vi "Inverter LUT UI.vi"(10 "Caller VI Refnum (Callee's Caller)":refnum<vi>, 11 "Main in":refnum<class "Main.lvclass">) -> (3 "Main out":refnum<class "Main.lvclass">)   [LabVIEW 2019, in "Main.lvclass"]
doc: "Developed by Kevin Thompson\nkevin@thompsonengineering.net\n\nCopyright 2020\nThompson Engineering, LLC"
uses:
  Main.lvclass
  Common/DataTypes/inverter info v2--cluster.ctl
  Common/DataTypes/inverter gain range--cluster.ctl
  Common/DataTypes/inverter offset range--cluster.ctl
  Common/DataTypes/Inverter database record v2--cluster.ctl
  Common/DataTypes/Inverter LUT v2--cluster.ctl
  <vilib>/TELLC/Dynamic CVT API/TD Dynamic CVT DVR--ref.ctl
  Main.lvclass/Main.ctl
  DataTypes/AsynCmd_Main--enum.ctl
  Accessors/Get InverterLUT Dict Ref.vi
  Accessors/Get ObjData.vi
  Accessors/Get Settings.vi
  Accessors/Set Settings.vi
  Accessors/Set InverterLUT Dict Ref.vi
  Accessors/Set CurrInverter Record.vi
  Config/Config.lvclass
  DAQ_Engine/DAQ_Engine.lvclass
  Log_Engine/Log_Engine.lvclass
panel:
  out "last updated":string="Micro < 500W"
  in  "offset range":T1={"offset max"=3000.0, "offset min"=2000.0, "offset increment"=0.0} caption="Offset Range"
  in  "gain range":T2={"gain max"=4000.0, "gain min"=3000.0, "gain increment"=100.0} caption="Gain Range"
  in  "resistance 3 phase":dbl
  in  "resistance single phase":dbl=50.0
  in  "minimum current":dbl
  in  "power level":dbl
  in  "set flag":u16(ring) items=["False", "True"]
  in  "gain actual":dbl
  in  "offset actual":dbl
  in  "inverter Info":T3
  in  "type":string="Micro < 500W"
  in  "name":string="Inverter-01"
  out "CurrRec":i32 caption="Current\nRecord Index"
  out "Total":i32 caption="Total Inverter\nRecords"
  in  "Inverter List":i32(listbox)
  in  "AddRec":bool
  in  "DeleteRec":bool
  in  "LUT File":path
  in  "Load":bool
  in  "UpdateRec":bool
  in  "Exit":bool
  # "Inverter Record"
  # "auto filled"
  # "INVERTER  DATABASE  EDITOR"
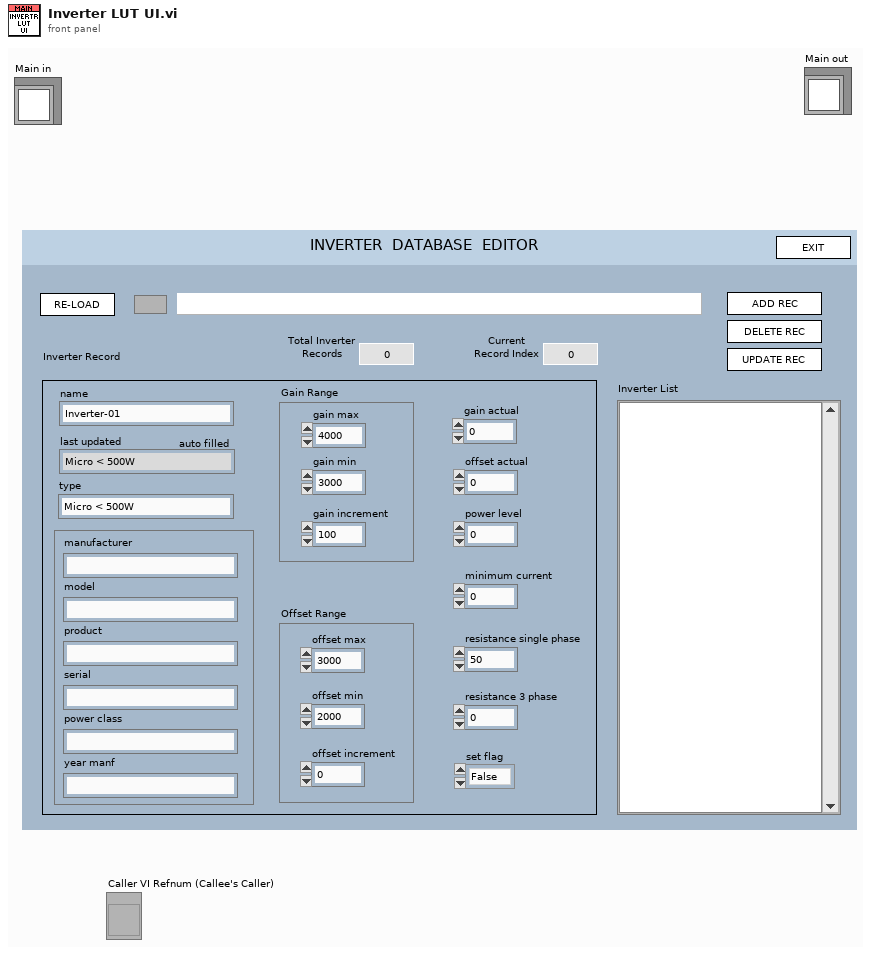
[diagram p1: front panel]
types:
  T1 = typedef "inverter offset range--cluster.ctl" = cluster{"offset max":dbl, "offset min":dbl, "offset increment":dbl}
  T2 = typedef "inverter gain range--cluster.ctl" = cluster{"gain max":dbl, "gain min":dbl, "gain increment":dbl}
  T3 = typedef "inverter info v2--cluster.ctl" = cluster{"manufacturer":string, "model":string, "product":string, "serial":string, "power class":string, "year manf":string}
  T4 = typedef "Inverter LUT v2--cluster.ctl" = cluster{"Inverter Records":T5[]}
  T5 = typedef "Inverter database record v2--cluster.ctl" = cluster{"name":string, "last updated":timestamp, "type":string, "inverter Info":T3, "gain range":T2, "offset range":T1, "gain actual":dbl, "offset actual":dbl, "power level":dbl, "minimum current":dbl, "resistance single phase":dbl, "resistance 3 phase":dbl, "set flag":u16}
  T6 = enum32{"invalid app kind", "Development System", "Run Time System", "Student Edition", "Embedded LabVIEW", "Evaluation", "Custom"}
  T7 = enum32{"Invalid", "Default", "Floating", "Floating/Auto-Hide", "Modal"}
  T8 = typedef "Main.lvclass/AsynCmd_Main--enum.ctl" = enum16{"Main.StartProcessing", "Main.StopProcessing", "Main.RefreshInverterList"}
  T9 = enum32{"Invalid", "Standard", "Closed", "Hidden", "Minimized", "Maximized"}
  T10 = typedef "TD Dynamic CVT DVR--ref.ctl" = refnum<data-value>
  T11 = cluster{"Core":cluster{"Current VI Reference":refnum<vi>, "Close Panel on Exit?":bool}, "CurrInverterRec":T5, "All Records":T5[], "Inverter Database File":path, "InverterLUT Dict":T10}
  T12 = cluster{"Current VI Reference":refnum<vi>, "Close Panel on Exit?":bool}
  T13 = typedef "Main.lvclass/ObjData--cluster.ctl" = cluster{"Settings":T14, "Public Events":T17, "Dependency":T18, "ReadData-placeholder":T19, "VISA-placeholder":refnum<visa-resource-name>, "InverterWaveformsQ":T20, "Application.TerminateProcess Event":refnum<user-event>, "RawDaqDataQ":T21, "MeasSettings":T22, "InverterDataAcqMode":T23, "DAQState Data":T24, "Private Events":T26, "InvWfmsQ-DT":T20, "DPAuxDataQ":T27, "ProcessingState":T28, "InverterInfo":T29, "CurrInverters":T5[], "InverterLUT Dict":T10, "ESR Chart Ref":refnum<vi>[], "StoreESR BLine Ref":refnum<vi>, "UseSavedESR BLine Ref":refnum<vi>, "CurrSensor":T30, "SensorLUT Dict":T10}
  T14 = typedef "Main.lvclass/Settings--cluster.ctl" = cluster{"Simulation":bool, "Signal scaling":T15[], "ESR scaling":T16[], "num readings to average":i32[], "ESR alarm threshhold (%)":i32[], "UseDummyVrms":bool, "Dummy Vrms":dbl, "Inverter Database File":path, "default Inverter (name)":string[], "Minimum Current Threshold ":dbl[], "Sensors Database File":path, "default Sensors (name)":string[]}
  T15 = typedef "Main.lvclass/Gain control.ctl" = cluster{"Iin ripple gain":dbl, "Iout ripple gain":dbl, "Iout 60Hz gain ":dbl, "Vout 60Hz gain ":dbl, "Iin ripple offest":dbl, "Iout ripple offset":dbl, "Iout 60Hz offset":dbl, "Vout 60Hz offset":dbl}
  T16 = typedef "Main.lvclass/ESR scaling--cluster.ctl" = cluster{"Gain":dbl, "Offset":dbl}
  T17 = typedef "Main.lvclass/Public Events--cluster.ctl" = cluster{"Main.AsyncCmd Event":refnum<user-event>, "Main.AsyncMsg Event":refnum<user-event>, "stop process":refnum<user-event>, "UpdateControlValue Ev":refnum<user-event>, "ProcessingStateChg Ev":refnum<user-event>}
  T18 = typedef "Main.lvclass/Dependency--cluster.ctl" = cluster{"Config":refnum<class "Config.lvclass">, "DAQ":refnum<class "DAQ_Engine.lvclass">, "Log_Engine":refnum<class "Log_Engine.lvclass">}
  T19 = typedef "Main.lvclass/Read Data--cluster.ctl" = cluster{"Data":dbl}
  T20 = typedef "InverterWaveforms--QRef.ctl" = refnum<queue>
  T21 = typedef "RawDAQDataQRef--cluster.ctl" = refnum<queue>
  T22 = typedef "Measurement Config--cluster.ctl" = cluster{"Data Rate 9775":dbl, "Data Rate 9215":dbl, "Samples RMS 9215":u32, "Samples RMS 9775":u32}
  T23 = typedef "Acquisition Mode--cluster.ctl" = enum16{"3phase", "Single"}
  T24 = typedef "DAQ_Engine.lvclass/DAQStateEvData--cluster.ctl" = cluster{"DAQState":T25, "vData":variant}
  T25 = typedef "DAQState--enum.ctl" = enum16{"Unknown", "Stopped", "Running", "Error"}
  T26 = typedef "Main.lvclass/Private Events--cluster.ctl" = cluster{"PrivateAsync Ev":refnum<user-event>}
  T27 = typedef "DataProcAuxDat--Qref.ctl" = refnum<queue>
  T28 = typedef "Main.lvclass/ProcessingState--enum.ctl" = enum16{"Idle", "Starting", "Running", "Done", "Error"}
  T29 = typedef "InverterInfo--cluster.ctl" = cluster{"Inverter ID":string}
  T30 = typedef "Sensor LUT--cluster.ctl" = T31[]
  T31 = typedef "Sensor database record--cluster.ctl" = cluster{"name":string, "last updated":timestamp, "manufacturer":string, "model":string, "Sensitivity index":dbl, "Sensor Ranges":T32}
  T32 = typedef "Sensor ranges--cluster.ctl" = cluster{"Max.VOut.RMS (V)":dbl, "Max.Out.Peak (V)":dbl, "Sensitivity (mV/A)":dbl, "Max.IOut.RMS(A)":dbl, "Min.IOut.RMS(A)":dbl}
  T33 = enum16{"Left Button", "Center Button", "Right Button", "Window Close"}
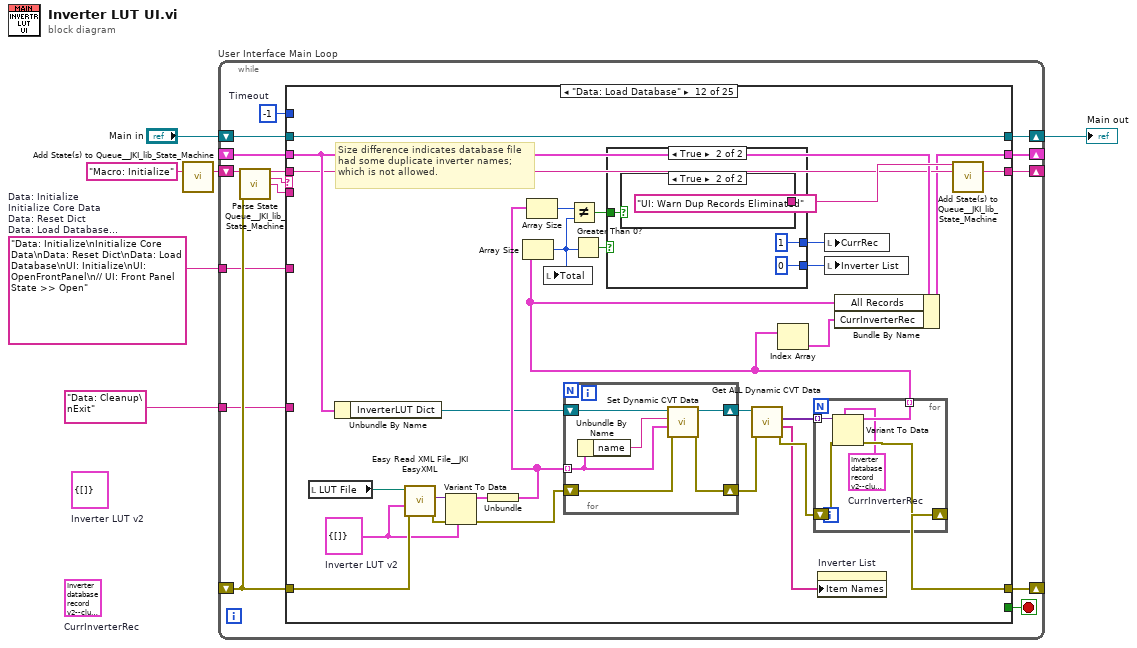
[diagram p0: block diagram]
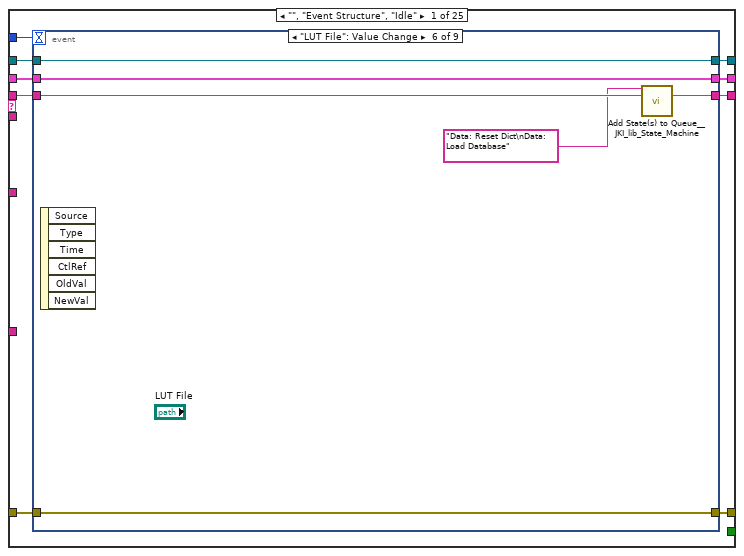
[diagram p2: hidden frame]
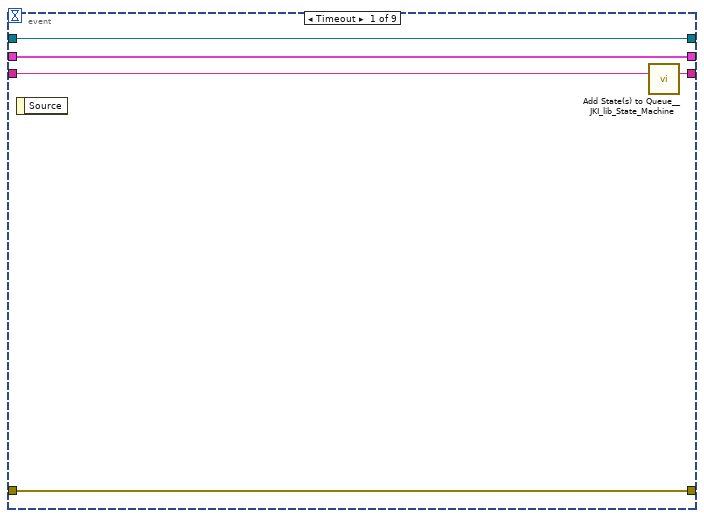
[diagram p3: hidden frame]
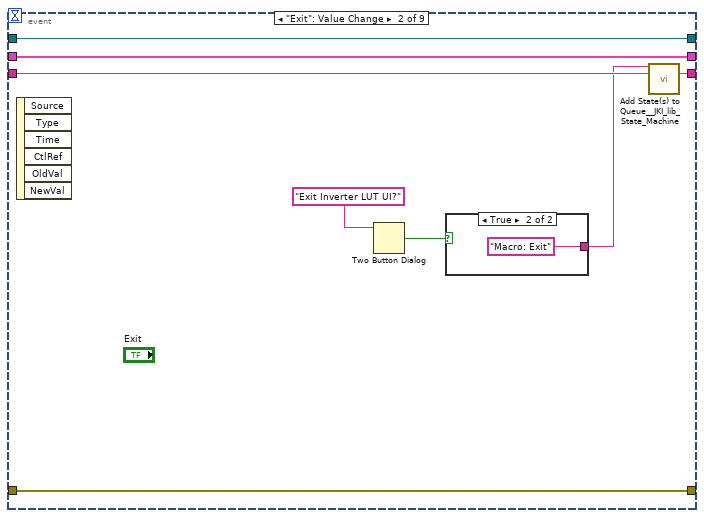
[diagram p4: hidden frame]
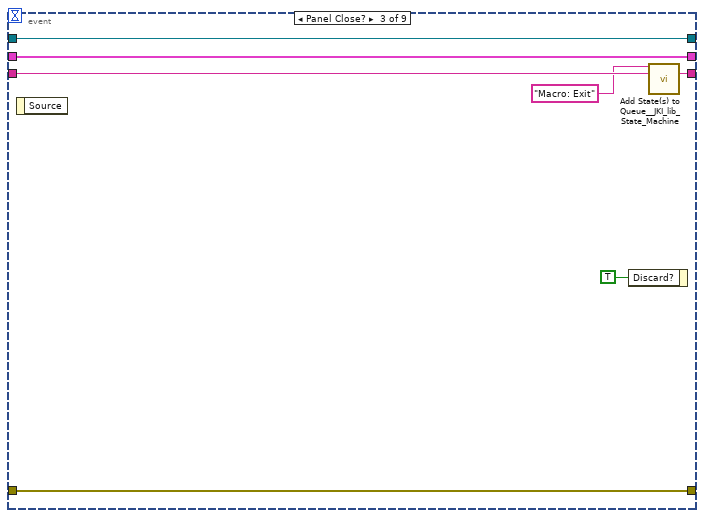
[diagram p6: hidden frame]
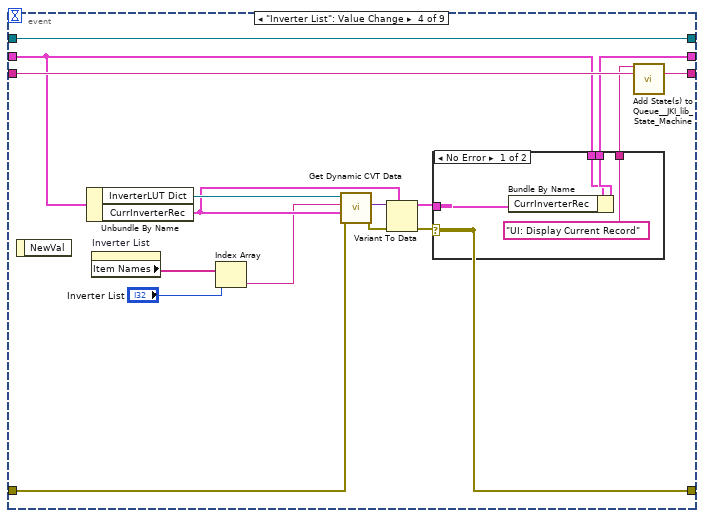
[diagram p7: hidden frame]
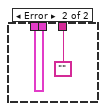
[diagram p8: hidden frame]
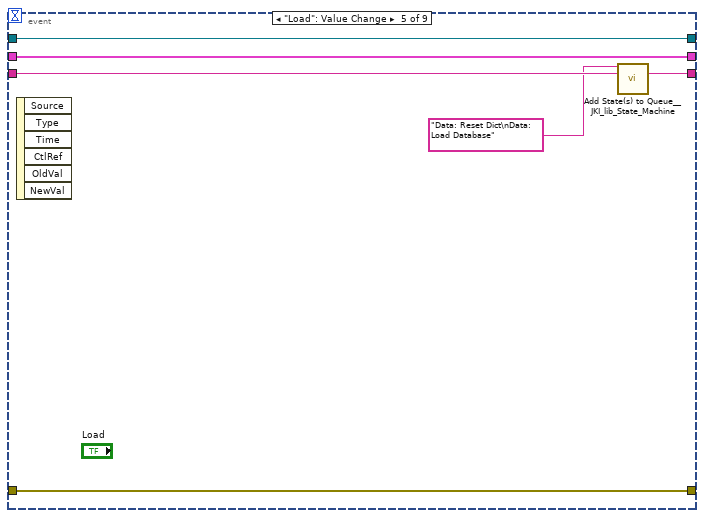
[diagram p9: hidden frame]
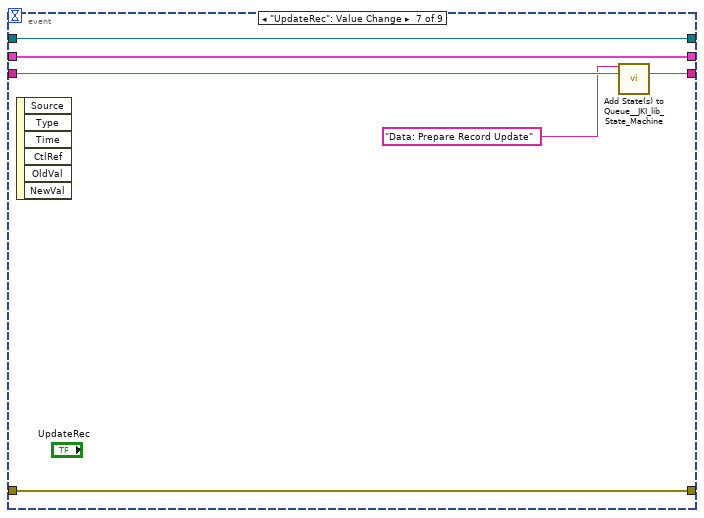
[diagram p10: hidden frame]
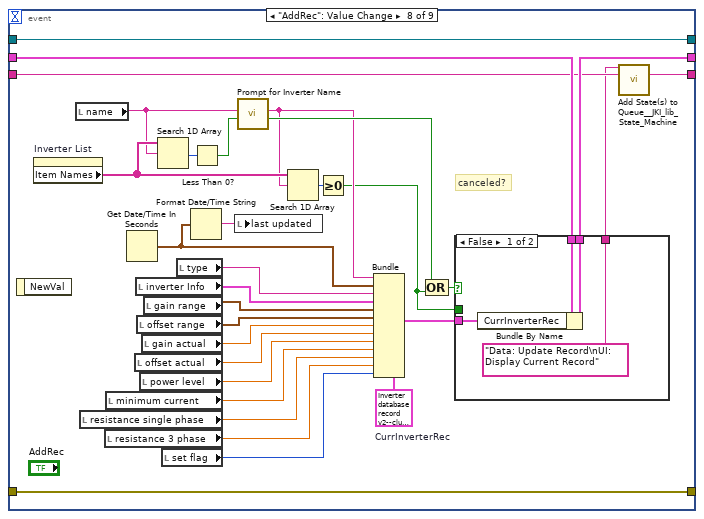
[diagram p11: hidden frame]
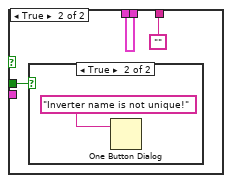
[diagram p12: hidden frame]
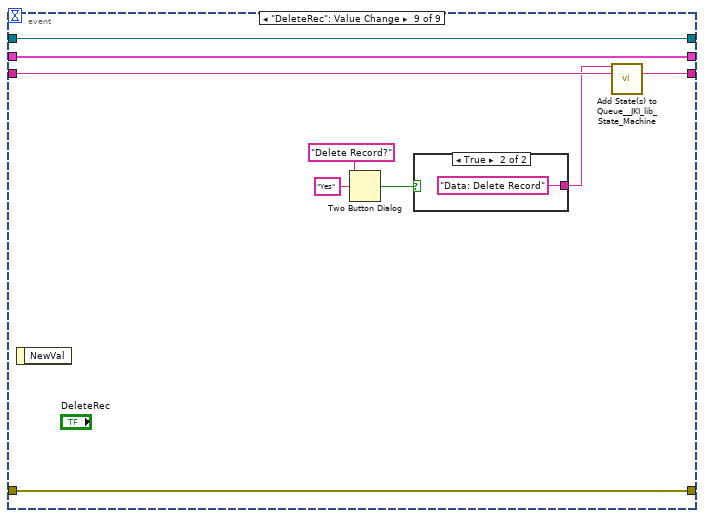
[diagram p14: hidden frame]
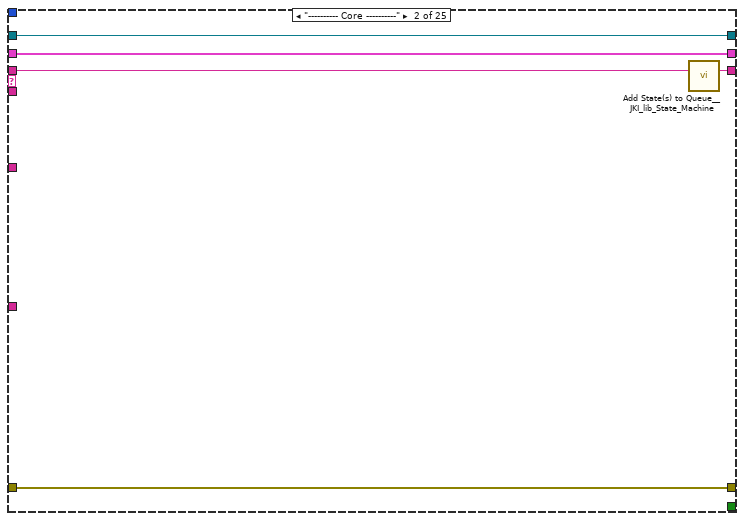
[diagram p16: hidden frame]
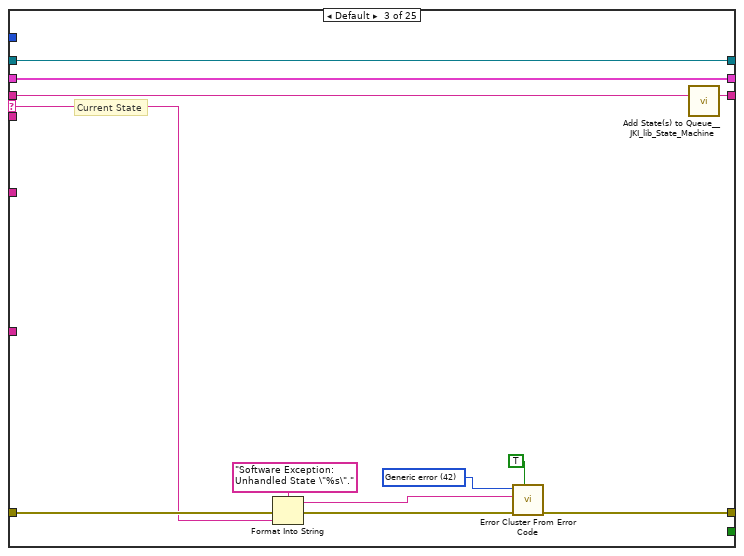
[diagram p17: hidden frame]
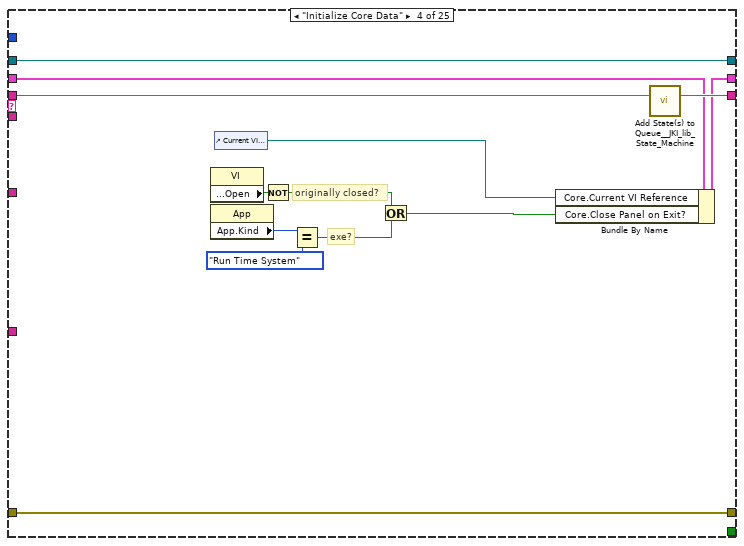
[diagram p18: hidden frame]
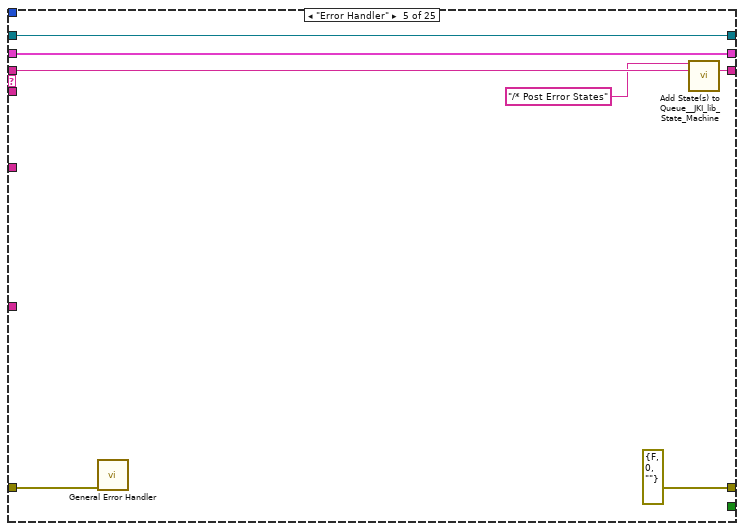
[diagram p19: hidden frame]
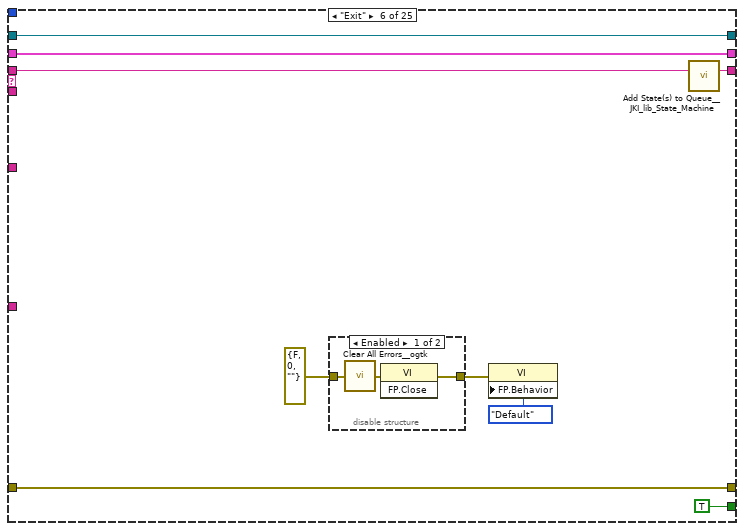
[diagram p20: hidden frame]
diagram:
  (unwired) T4 {"Inverter Records"=[]}  # Inverter LUT v2
  (unwired) T5 {"name"="", "last updated"=timestamp(0 s since 1904-01-01), "type"="", "inverter Info"={"manufacturer"="", "model"="", "product"="", "serial"="", "power class"="", "year manf"=""}, "gain range"={"gain max"=0.0, "gain min"=0.0, "gain increment"=0.0}, "offset range"={"offset max"=0.0, "offset min"=0.0, "offset increment"=0.0}, "gain actual"=0.0, "offset actual"=0.0, "power level"=0.0, "minimum current"=0.0, "resistance single phase"=0.0, "resistance 3 phase"=0.0, "set flag"=0}  # CurrInverterRec
  w4 = "Data: Initialize\nInitialize Core Data\nData: Reset Dict\nData: Load Database\nUI: Initialize\nUI: OpenFrontPanel\n// UI: Front Panel State >> Open"  # Data: Initialize Initialize Core Data Data: Reset Dict Data: Load Database UI: Initialize UI: OpenFrontPanel // UI: Front Panel State >> Open
  n1 = call <vilib>:"Add State(s) to Queue__JKI_lib_State_Machine.vi"("State(s) in (\"\")"="Macro: Initialize") -> ("States Out"=w6:string)  [unwired: 14 in]
  n2 = while "User Interface Main Loop" {
    shift-right: [w14] -> _
    shift-left: _ -> [w13]
    shift-right: [w17] -> _
    shift-left: _ -> [w11]
    shift-right: [w16] -> _
    shift-left: w6 -> [w18]
    tunnel: w4 -> [w10]
    tunnel: "Data: Cleanup\nExit" -> [w9]
    shift-right: [w7] -> w1
    shift-left: "Main in" -> [w8]
    stop <- w15 stop-if-true
    w12 = -1  # Timeout
    n3 = call <vilib>:"Parse State Queue__JKI_lib_State_Machine.vi"("State Queue"=w18, "Error In (no error)"=w11) -> ("Remaining States"=w20:string, "Current State"=w21:string, "Arguments"=w19:string)  [unwired: 11 in]
    n4 = case shown="\"Data: Load Database\"" w21 {
      selector: w21 -> [_ _ w147 _ _ _ _ _ _ _ _ _ _ _ _ _ _ _ _ _ _ _ _ _ _]
      tunnel: w20 -> [w30 w145 w151 w170 w177 w186 w195 w224 w237 w258 w288 w299 w363 w386 w401 w411 w436 w459 w479 w486 w498 w525 w531 w542 w547]
      tunnel: w19 -> [_ _ _ _ _ _ _ _ _ _ _ _ _ _ _ _ _ _ _ w481 w492 _ _ _ _]
      tunnel: w13 -> [w28 w142 w149 w161 w174 w184 w192 w218 w235 w248 w286 w306 _ w374 w398 w408 w422 w444 w471 w484 w494 w522 w528 w539 w544]
      tunnel: [w27 w143 w153 w167 errorcluster {"status"=FALSE, "code"=0, "source"=""} ("error out") w183 w193 w222 w233 w243 w277 w301 w360 w382 w399 w409 w434 w457 w461 w482 w495 w523 w529 w540 w545] -> w17
      tunnel: w11 -> [w26 w143 w152 w167 w173 w183 w193 w222 w232 w242 w283 w302 w360 w383 w399 w409 w434 w457 w468 w483 w496 w523 w529 w540 w545]
      tunnel: [w29 w144 w150 w169 w176 w185 w194 w223 w236 w257 w287 w300 w362 w385 w400 w410 w435 w458 w478 w485 w497 w524 w530 w541 w546] -> w16
      tunnel: [_ _ _ _ _ TRUE _ _ _ _ _ _ _ _ _ _ _ _ _ _ _ _ _ _ _] -> w15
      tunnel: [w25 w142 w149 w168 w174 w184 w192 w217 w235 w249 w286 w298 w361 w374 w398 w408 w422 w444 w471 w484 w494 w522 w528 w539 w544] -> w14
      tunnel: w12 -> [w24 _ _ _ _ _ _ _ _ _ _ _ _ _ _ _ _ _ _ _ _ _ _ _ _]
      tunnel: w10 -> [_ _ _ _ _ _ _ _ _ _ _ _ _ _ _ _ _ _ _ _ _ _ w527 _ _]
      tunnel: w9 -> [_ _ _ _ _ _ _ _ _ _ _ _ _ _ _ _ _ _ _ _ _ _ _ w533 _]
      tunnel: w8 -> [w23 w141 w146 w158 w171 w178 w191 w211 w231 w240 w267 w323 w350 w379 w397 w407 w417 w439 w462 w480 w491 w521 w526 w532 w543]
      tunnel: [w22 w141 w146 w158 w171 w178 w191 w211 w231 w240 w267 w323 w351 w365 w397 w407 w417 w439 w462 w480 w491 w521 w526 w532 w543] -> w7
      frame "", "Event Structure", "Idle" {
        n5 = event shown="[5] \"LUT File\": Value Change" {
          selector: _ -> [_ _ _ _ _ _ _ _ _]
          dyn-events: _ -> [_ _ _ _ _ _ _ _ _]
          timeout: w24 -> [_ _ _ _ _ _ _ _ _]
          tunnel: w30 -> [w35 w43 w51 w60 w76 w83 w89 w117 w134]
          tunnel: [w34 w42 w50 w61 w77 w84 w90 w118 w135] -> w29
          tunnel: w28 -> [w32 w40 w48 w57 w78 w81 w88 w120 w138]
          tunnel: [w33 w41 w49 w55 w79 w85 w91 w122 w139] -> w27
          tunnel: w26 -> [w33 w41 w49 w54 w79 w85 w91 w122 w139]
          tunnel: [w32 w40 w48 w58 w78 w81 w88 w121 w138] -> w25
          tunnel: [w31 w36 w45 w53 w74 w80 w86 w115 w131] -> w22
          tunnel: w23 -> [w31 w36 w45 w53 w74 w80 w86 w115 w131]
          event Timeout {
            n6 = event-data() -> ()  [unwired: 1 in, 1 out]
            n7 = call <vilib>:"Add State(s) to Queue__JKI_lib_State_Machine.vi"("State(s) in (\"\")"=w35) -> ("States Out"=w34:string)  [unwired: 14 in]
          }
          event "Exit": Value Change {
            n8 = event-data() -> ()  [unwired: 1 in, 6 out]
            n9 = Two Button Dialog(message="Exit Inverter LUT UI?") -> (T button?=w37:bool)  [unwired: 2 in]
            n10 = case shown="True" w37 {
              tunnel: [_ "Macro: Exit"] -> w39
              frame False {
              }
              frame True {
              }
            }
            n11 = call <vilib>:"Add State(s) to Queue__JKI_lib_State_Machine.vi"("State(s) in Front (\"\")"=w39, "State(s) in (\"\")"=w43) -> ("States Out"=w42:string)  [unwired: 13 in]
          }
          event Panel Close? {
            n12 = event-data() -> ()  [unwired: 1 in, 1 out]
            n13 = event-data("Discard?"=TRUE) -> ()  [unwired: 1 in, 1 out]
            n14 = call <vilib>:"Add State(s) to Queue__JKI_lib_State_Machine.vi"("State(s) in Front (\"\")"="Macro: Exit", "State(s) in (\"\")"=w51) -> ("States Out"=w50:string)  [unwired: 13 in]
          }
          event "Inverter List": Value Change {
            n15 = event-data() -> ()  [unwired: 1 in, 1 out]
            n16 = Unbundle By Name(w57) -> ("InverterLUT Dict"=w65:T10, "CurrInverterRec"=w63:T5)
            n17 = property on="Inverter List" class="LstBox (strict)"() -> ("Item Names"=w67:string[])  [unwired: 2 in, 2 out]
            n18 = Index Array(array=w67, index="Inverter List") -> (element=w52:string)
            n19 = call <vilib>:"Get Dynamic CVT Data.vi"("error in (no error)"=w54, "default value (empty variant)"=w63, "DataName"=w52, "dCVT DVR"=w65) -> ("error out"=w64:errorcluster, "value"=w62:variant)  [unwired: 4 in, 2 out]
            n20 = Variant To Data(error in=w64, type=w63, Variant=w62) -> (data=w59:T5, error out=w55:errorcluster)
            n21 = case shown="No Error" w55 {
              tunnel: w59 -> [w68 _]
              tunnel: [w71 w73] -> w58
              tunnel: w57 -> [w70 w73]
              tunnel: ["UI: Display Current Record" ""] -> w56
              frame No Error {
                n22 = Bundle By Name(cluster=w70, "CurrInverterRec"=w68) -> (w71:T11)
              }
              frame Error {
              }
            }
            n23 = call <vilib>:"Add State(s) to Queue__JKI_lib_State_Machine.vi"("State(s) in Front (\"\")"=w56, "State(s) in (\"\")"=w60) -> ("States Out"=w61:string)  [unwired: 13 in]
          }
          event "Load": Value Change {
            n24 = event-data() -> ()  [unwired: 1 in, 6 out]
            n25 = call <vilib>:"Add State(s) to Queue__JKI_lib_State_Machine.vi"("State(s) in Front (\"\")"="Data: Reset Dict\nData: Load Database", "State(s) in (\"\")"=w76) -> ("States Out"=w77:string)  [unwired: 13 in]
          }
          event "LUT File": Value Change {
            n26 = event-data() -> ()  [unwired: 1 in, 6 out]
            n27 = call <vilib>:"Add State(s) to Queue__JKI_lib_State_Machine.vi"("State(s) in Front (\"\")"="Data: Reset Dict\nData: Load Database", "State(s) in (\"\")"=w83) -> ("States Out"=w84:string)  [unwired: 13 in]
          }
          event "UpdateRec": Value Change {
            n28 = event-data() -> ()  [unwired: 1 in, 6 out]
            n29 = call <vilib>:"Add State(s) to Queue__JKI_lib_State_Machine.vi"("State(s) in Front (\"\")"="Data: Prepare Record Update", "State(s) in (\"\")"=w89) -> ("States Out"=w90:string)  [unwired: 13 in]
          }
          event "AddRec": Value Change {
            w114 = T5 {"name"="", "last updated"=timestamp(0 s since 1904-01-01), "type"="", "inverter Info"={"manufacturer"="", "model"="", "product"="", "serial"="", "power class"="", "year manf"=""}, "gain range"={"gain max"=0.0, "gain min"=0.0, "gain increment"=0.0}, "offset range"={"offset max"=0.0, "offset min"=0.0, "offset increment"=0.0}, "gain actual"=0.0, "offset actual"=0.0, "power level"=0.0, "minimum current"=0.0, "resistance single phase"=0.0, "resistance 3 phase"=0.0, "set flag"=0}  # CurrInverterRec
            # "canceled?"
            n30 = event-data() -> ()  [unwired: 1 in, 1 out]
            n31 = property on="Inverter List" class="LstBox (strict)"() -> ("Item Names"=w98:string[])  [unwired: 2 in, 2 out]
            n32 = local read "name"() -> (w92:string)
            n33 = local read "resistance single phase"() -> (w111:dbl)
            n34 = local read "resistance 3 phase"() -> (w112:dbl)
            n35 = local read "minimum current"() -> (w110:dbl)
            n36 = Get Date/Time In Seconds() -> (seconds since 1Jan1904=w102:timestamp)
            n37 = local read "offset actual"() -> (w108:dbl)
            n38 = local read "inverter Info"() -> (w104:T3)
            n39 = local read "offset range"() -> (w106:T1)
            n40 = local read "power level"() -> (w109:dbl)
            n41 = local read "gain actual"() -> (w107:dbl)
            n42 = local read "gain range"() -> (w105:T2)
            n43 = Search 1D Array(1D array=w98, element=w92) -> (index of element=w99:i32)  [unwired: 1 in]
            n44 = local read "set flag"() -> (w113:u16)
            n45 = local read "type"() -> (w103:string)
            n46 = Format Date/Time String(seconds (now)=w102) -> (date/time string=w101:string)  [unwired: 2 in]
            n47 = Less Than 0?(x=w99) -> (x < 0?=w97:bool)
            n48 = local write "last updated"(w101) -> ()
            n49 = call "Prompt for Inverter Name.vi"("bypass (F)"=w97, "Name"=w92) -> ("canceled"=w96:bool, "name out"=w95:string)  [unwired: 7 in, 1 out]
            n50 = Search 1D Array(1D array=w98, element=w95) -> (index of element=w100:i32)  [unwired: 1 in]
            n51 = Greater Or Equal To 0?(x=w100) -> (x >= 0?=w94:bool)
            n52 = Bundle(cluster=w114, "name"=w95, "last updated"=w102, "type"=w103, "inverter Info"=w104, "gain range"=w105, "offset range"=w106, "gain actual"=w107, "offset actual"=w108, "power level"=w109, "minimum current"=w110, "resistance single phase"=w111, "resistance 3 phase"=w112, "set flag"=w113) -> (w119:T5)
            n53 = Compound Arithmetic op=OR(w96, w94) -> (w93:bool)
            n54 = case shown="False" w93 {
              tunnel: [w126 w129] -> w121
              tunnel: w120 -> [w125 w129]
              tunnel: w119 -> [w124 _]
              tunnel: ["Data: Update Record\nUI: Display Current Record" ""] -> w116
              tunnel: w94 -> [_ w127]
              frame False {
                n55 = Bundle By Name(cluster=w125, "CurrInverterRec"=w124) -> (w126:T11)
              }
              frame True {
                n56 = case shown="True" w127 {
                  frame False {
                  }
                  frame True {
                    n57 = One Button Dialog(message="Inverter name is not unique!") -> ()  [unwired: 1 in, 1 out]
                  }
                }
              }
            }
            n58 = call <vilib>:"Add State(s) to Queue__JKI_lib_State_Machine.vi"("State(s) in Front (\"\")"=w116, "State(s) in (\"\")"=w117) -> ("States Out"=w118:string)  [unwired: 13 in]
          }
          event "DeleteRec": Value Change {
            n59 = event-data() -> ()  [unwired: 1 in, 1 out]
            n60 = Two Button Dialog(message="Delete Record?", 2:"Yes" ("T button name (\"OK\")")) -> (T button?=w132:bool)  [unwired: 1 in]
            n61 = case shown="True" w132 {
              tunnel: [_ "Data: Delete Record"] -> w133
              frame False {
              }
              frame True {
              }
            }
            n62 = call <vilib>:"Add State(s) to Queue__JKI_lib_State_Machine.vi"("State(s) in Front (\"\")"=w133, "State(s) in (\"\")"=w134) -> ("States Out"=w135:string)  [unwired: 13 in]
          }
        }
      }
      frame "---------- Core ----------" {
        n63 = call <vilib>:"Add State(s) to Queue__JKI_lib_State_Machine.vi"("State(s) in (\"\")"=w145) -> ("States Out"=w144:string)  [unwired: 14 in]
      }
      frame Default {
        w156 = 42 items=["No error", "Argument error", "Memory is full", "Out of zone", "End of file", "File already open", "Generic file I/O error", "File not found", "File permission error", "Disk is full", "Duplicate path", "Too many files open", "System feature not enabled", "Resource file not found", "Cannot add resource", "Resource not found", "Image not found", "Image memory error", "Pen does not exist", "Config type invalid", "Config token not found", "Config parse error", "Config memory error", "Bad external code format", "Bad external code offset", "External code not present", "Null window", "Destroy window error", "Null menu", "Print aborted", "Bad print record", "Print driver error", "Windows error during printing", "Memory error during printing", "Print dialog error", "Generic print error", "Invalid device refnum", "Device not found", "Device parameter error", "Device unit error", "Cannot open device", "Device call aborted", "Generic error", "Cancelled by user", "Object ID too low", "Object ID too high", "Object not in heap", "Unknown heap", "Unknown object (invalid DefProc)", "Unknown object (DefProc not in table)", "Message out of range", "Invalid (null) method", "Unknown message", "Manager call not supported", "Bad address", "Network operation in progress", "Network operation timed out", "Connection is busy", "Network attribute not supported", "Network error", "Address in use", "System out of memory", "Connection aborted", "Connection refused", "Not connected", "Already connected", "Connection closed", "Initialization error (interapplication manager)", "Bad occurrence", "Wait on unbound occurrence handler", "Occurrence queue overflow", "Datalog type conflict", "Unused", "Unrecognized type (interapplication manager)", "Memory corrupt", "Failed to make temporary DLL", "Old CIN version", "Drag socket not found", "Failed to load drop-object", "Failed to register OLE object", "Failed to release OLE object", "Format specifier type mismatch", "Unknown format specifier", "Too few format specifiers", "Too many format specifiers", "Scan failed", "Newer CIN version", "Error converting to variant", "Runtime menu error", "Password tampered", "Variant attribute not found", "Incompatible variant data type", "Event data is not available", "Event Store is not present", "Occurrence is not found", "Event Queue is not created", "Event info is not available", "Refnum passed is NULL", "Error retrieving Class GUID", "Error retrieving CoClass GUID", "Error retrieving TypeLib GUID.", "Bad built application magic bytes.", "Specific driver is different from the specific driver associated with the Logical Name.", "There is no session opened to the class driver.", "Max Error", "MAX - Error with config objects", "MAX - Error loading configuration", "MAX - Group not supported"]
        # "Current State"
        n64 = Format Into String(format string="Software Exception: Unhandled State \"%s\"." ("message"), error in=w152, w147) -> (resulting string=w155:string, error out=w154:errorcluster)  [unwired: 1 in]
        n65 = call <vilib>:"Error Cluster From Error Code.vi"("show call chain? (False)"=TRUE, "error in (no error)"=w154, "error message (\"\")"=w155, "error code (0)"=w156) -> ("error out"=w153:errorcluster)  [unwired: 5 in]
        n66 = call <vilib>:"Add State(s) to Queue__JKI_lib_State_Machine.vi"("State(s) in (\"\")"=w151) -> ("States Out"=w150:string)  [unwired: 14 in]
      }
      frame "Initialize Core Data" {
        # "originally closed?"
        # "exe?"
        n67 = property class="VI"() -> ("Front Panel.Open"=w166:bool)  [unwired: 2 in, 2 out]
        n68 = property class="App"() -> ("App.Kind"=w165:T6)  [unwired: 2 in, 2 out]
        n69 = control-ref of="Current VI Reference"() -> (w159:refnum<vi>)
        n70 = Not(x=w166) -> (.not. x?=w163:bool)
        n71 = Equal?(x=w165, y=T6."Run Time System" ("Application:Kind")) -> (x = y?=w162:bool)
        n72 = Or(x=w163, y=w162) -> (x .or. y?=w160:bool)
        n73 = Bundle By Name(cluster=w161, "Core.Current VI Reference"=w159, "Core.Close Panel on Exit?"=w160) -> (w168:T11)
        n74 = call <vilib>:"Add State(s) to Queue__JKI_lib_State_Machine.vi"("State(s) in (\"\")"=w170) -> ("States Out"=w169:string)  [unwired: 14 in]
      }
      frame "Error Handler" {
        n75 = call <vilib>:"General Error Handler.vi"("error in (no error)"=w173) -> ()  [unwired: 10 in, 5 out]
        n76 = call <vilib>:"Add State(s) to Queue__JKI_lib_State_Machine.vi"("State(s) in Front (\"\")"="/* Post Error States", "State(s) in (\"\")"=w177) -> ("States Out"=w176:string)  [unwired: 13 in]
      }
      frame "Exit" {
        n77 = disable-structure shown="Enabled" {
          disable-tunnel: [w189 w190] -> w181
          disable-tunnel: errorcluster {"status"=FALSE, "code"=0, "source"=""} ("Error In") -> [w187 w190]
          frame Enabled {
            n78 = call <userlib>:"Clear All Errors__ogtk.vi"("Error In"=w187) -> ("Error Out"=w188:errorcluster)  [unwired: 3 in]
            n79 = invoke class="VI" method="FP.Close"(error in=w188) -> (error out=w189:errorcluster)  [unwired: 2 in, 2 out]
          }
          frame Disabled {
          }
        }
        n80 = property class="VI"(error in=w181, "FP.Behavior"=T7."Default" ("Front Panel Window:Behavior")) -> ()  [unwired: 1 in, 2 out]
        n81 = call <vilib>:"Add State(s) to Queue__JKI_lib_State_Machine.vi"("State(s) in (\"\")"=w186) -> ("States Out"=w185:string)  [unwired: 14 in]
      }
      frame "---------- Data ----------" {
        n82 = call <vilib>:"Add State(s) to Queue__JKI_lib_State_Machine.vi"("State(s) in (\"\")"=w195) -> ("States Out"=w194:string)  [unwired: 14 in]
      }
      frame "Data: Prepare Record Update" {
        w210 = T5 {"name"="", "last updated"=timestamp(0 s since 1904-01-01), "type"="", "inverter Info"={"manufacturer"="", "model"="", "product"="", "serial"="", "power class"="", "year manf"=""}, "gain range"={"gain max"=0.0, "gain min"=0.0, "gain increment"=0.0}, "offset range"={"offset max"=0.0, "offset min"=0.0, "offset increment"=0.0}, "gain actual"=0.0, "offset actual"=0.0, "power level"=0.0, "minimum current"=0.0, "resistance single phase"=0.0, "resistance 3 phase"=0.0, "set flag"=0}  # CurrInverterRec
        # "Update Record only updates record values; it does not add a new record."
        n83 = local read "Inverter List"() -> (w215:i32)
        n84 = property on="Inverter List" class="LstBox (strict)"() -> ("Item Names"=w214:string[])  [unwired: 2 in, 2 out]
        n85 = Get Date/Time In Seconds() -> (seconds since 1Jan1904=w196:timestamp)
        n86 = Index Array(array=w214, index=w215) -> (element=w198:string)
        n87 = Format Date/Time String(seconds (now)=w196) -> (date/time string=→"last updated":string)  [unwired: 2 in]
        n88 = local write "name"(w198) -> ()
        n89 = Format Into String(format string="Update Record for [%s] in Database File?\n(Use ADD REC button to add new record.)" ("message"), w198) -> (resulting string=w212:string)  [unwired: 2 in, 1 out]
        n90 = Two Button Dialog(message=w212, 2:"Yes" ("T button name (\"OK\")")) -> (T button?=w220:bool)  [unwired: 1 in]
        n91 = Bundle(cluster=w210, "name"=w198, "last updated"=w196, "type"="type", "inverter Info"="inverter Info", "gain range"="gain range", "offset range"="offset range", "gain actual"="gain actual", "offset actual"="offset actual", "power level"="power level", "minimum current"="minimum current", "resistance single phase"="resistance single phase", "resistance 3 phase"="resistance 3 phase", "set flag"="set flag") -> (w221:T5)
        n92 = case shown="True" w220 {
          tunnel: [w226 w230] -> w217
          tunnel: w218 -> [w226 w229]
          tunnel: w221 -> [_ w228]
          tunnel: ["" "Data: Update Record"] -> w216
          frame False {
          }
          frame True {
            n93 = Bundle By Name(cluster=w229, "CurrInverterRec"=w228) -> (w230:T11)
          }
        }
        n94 = call <vilib>:"Add State(s) to Queue__JKI_lib_State_Machine.vi"("State(s) in Front (\"\")"=w216, "State(s) in (\"\")"=w224) -> ("States Out"=w223:string)  [unwired: 13 in]
      }
      frame "Data: Reset Dict" {
        n95 = Unbundle By Name(w235) -> ("InverterLUT Dict"=w234:T10)
        n96 = call <vilib>:"Delete ALL Dynamic CVT Data.vi"("error in (no error)"=w232, "dCVT DVR"=w234) -> ("error out"=w233:errorcluster)  [unwired: 8 in, 1 out]
        n97 = call <vilib>:"Add State(s) to Queue__JKI_lib_State_Machine.vi"("State(s) in (\"\")"=w237) -> ("States Out"=w236:string)  [unwired: 14 in]
      }
      frame "Data: Delete Record" {
        w239 = T5 {"name"="", "last updated"=timestamp(0 s since 1904-01-01), "type"="", "inverter Info"={"manufacturer"="", "model"="", "product"="", "serial"="", "power class"="", "year manf"=""}, "gain range"={"gain max"=0.0, "gain min"=0.0, "gain increment"=0.0}, "offset range"={"offset max"=0.0, "offset min"=0.0, "offset increment"=0.0}, "gain actual"=0.0, "offset actual"=0.0, "power level"=0.0, "minimum current"=0.0, "resistance single phase"=0.0, "resistance 3 phase"=0.0, "set flag"=0}  # CurrInverterRec
        n98 = Unbundle By Name(w248) -> ("InverterLUT Dict"=w256:T10, "CurrInverterRec"=w254:T5)
        n99 = Unbundle By Name(w254) -> ("name"=w255:string)
        n100 = call <vilib>:"Delete Dynamic CVT Data.vi"("error in (no error)"=w242, "DataName"=w255, "dCVT DVR"=w256) -> ("error out"=w252:errorcluster, "CVT DVR out"=w253:T10)  [unwired: 6 in, 1 out]
        n101 = call <vilib>:"Get ALL Dynamic CVT Data.vi"("error in (no error)"=w252, "dCVT DVR"=w253) -> ("error out"=w245:errorcluster, "NameArray"=w250:string[], "ValueArray"=w251:variant[])  [unwired: 6 in, 1 out]
        n102 = Index Array(array=w251) -> (element=w238:variant)  [unwired: 1 in]
        n103 = property on="Inverter List" class="LstBox (strict)"(error in=w245, "Item Names"=w250) -> (error out=w246:errorcluster)  [unwired: 1 in, 1 out]
        n104 = Variant To Data(error in=w245, type=w239, Variant=w238) -> (data=w247:T5, error out=w244:errorcluster)
        n105 = Bundle By Name(cluster=w248, "CurrInverterRec"=w247) -> (w249:T11)
        n106 = flat-sequence {
          tunnel: w246 -> [w261]
          tunnel: w244 -> [w260]
          tunnel: [w259] -> w243
          frame #0 {
            n107 = Merge Errors(w260, w261) -> (w259:errorcluster)
            n108 = local write "Inverter List"(0 ("Inverter List")) -> ()
          }
        }
        n109 = call <vilib>:"Add State(s) to Queue__JKI_lib_State_Machine.vi"("State(s) in Front (\"\")"="Data: Update Record\nUI: Display Current Record", "State(s) in (\"\")"=w258) -> ("States Out"=w257:string)  [unwired: 13 in]
      }
      frame "Data: Update Record" {
        w266 = T5 {"name"="", "last updated"=timestamp(0 s since 1904-01-01), "type"="", "inverter Info"={"manufacturer"="", "model"="", "product"="", "serial"="", "power class"="", "year manf"=""}, "gain range"={"gain max"=0.0, "gain min"=0.0, "gain increment"=0.0}, "offset range"={"offset max"=0.0, "offset min"=0.0, "offset increment"=0.0}, "gain actual"=0.0, "offset actual"=0.0, "power level"=0.0, "minimum current"=0.0, "resistance single phase"=0.0, "resistance 3 phase"=0.0, "set flag"=0}  # CurrInverterRec
        n110 = Unbundle By Name(w286) -> ("InverterLUT Dict"=w285:T10, "CurrInverterRec"=w284:T5)
        n111 = Unbundle By Name(w284) -> ("name"=w275:string)
        n112 = call <vilib>:"Set Dynamic CVT Data.vi"("error in (no error)"=w283, "value"=w284, "DataName"=w275, "dCVT DVR"=w285) -> ("error out"=w281:errorcluster, "dCVT DVR out"=w282:T10)  [unwired: 5 in, 1 out]
        n113 = call <userlib>:"Clear All Errors__ogtk.vi"("Error In"=w281) -> ("Error Out"=w269:errorcluster)  [unwired: 3 in]
        n114 = call <vilib>:"Get ALL Dynamic CVT Data.vi"("error in (no error)"=w269, "dCVT DVR"=w282) -> ("error out"=w278:errorcluster, "NameArray"=w276:string[], "ValueArray"=w280:variant[])  [unwired: 6 in, 1 out]
        n115 = Index Array(array=w280) -> (element=w263:variant)  [unwired: 1 in]
        n116 = call <userlib>:"Clear All Errors__ogtk.vi"("Error In"=w278) -> ("Error Out"=w268:errorcluster)  [unwired: 3 in]
        n117 = Variant To Data(type=w266, Variant=w263) -> (data=w279:T5)  [unwired: 1 in, 1 out]
        n118 = Array Size(array=w276) -> (size(s)=→"Total":i32)
        n119 = Search 1D Array(1D array=w276, element=w275) -> (index of element=w274:i32)  [unwired: 1 in]
        n120 = property on="Inverter List" class="LstBox (strict)"("Item Names"=w276) -> ()  [unwired: 2 in, 2 out]
        n121 = local write "Inverter List"(w274) -> ()
        n122 = Variant To Data(type=T5 {"name"="", "last updated"=timestamp(0 s since 1904-01-01), "type"="", "inverter Info"={"manufacturer"="", "model"="", "product"="", "serial"="", "power class"="", "year manf"=""}, "gain range"={"gain max"=0.0, "gain min"=0.0, "gain increment"=0.0}, "offset range"={"offset max"=0.0, "offset min"=0.0, "offset increment"=0.0}, "gain actual"=0.0, "offset actual"=0.0, "power level"=0.0, "minimum current"=0.0, "resistance single phase"=0.0, "resistance 3 phase"=0.0, "set flag"=0} ("CurrInverterRec"), Variant=w279) -> (data=w264:T5)  [unwired: 1 in, 1 out]
        n123 = local read "LUT File"() -> (w271:path)
        n124 = Empty String/Path?(string/path=w271) -> (empty?=w270:bool)
        n125 = Increment(x=w274) -> (x+1=→"CurrRec":i32)
        n126 = case shown="False" w270 {
          tunnel: w264 -> [w293 _]
          tunnel: w268 -> [w291 w294]
          tunnel: [w290 w294] -> w277
          tunnel: w271 -> [w289 _]
          frame False {
            n127 = call <vilib>:"Easy Write XML File__JKI EasyXML.vi"("error in (no error)"=w291, "Overwrite File? (false)"=TRUE, "LabVIEW Data"=w293, "XML File Path"=w289) -> ("error out"=w290:errorcluster)  [unwired: 6 in, 1 out]
          }
          frame True {
          }
        }
        n128 = call <vilib>:"Add State(s) to Queue__JKI_lib_State_Machine.vi"("State(s) in (\"\")"=w288) -> ("States Out"=w287:string)  [unwired: 14 in]
      }
      frame "Data: Load Database" {
        w297 = T4 {"Inverter Records"=[]}  # Inverter LUT v2
        # "Size difference indicates database file\nhad some duplicate inverter names;\nwhich is not allowed."
        n129 = local read "LUT File"() -> (w319:path)
        n130 = Unbundle By Name(w306) -> ("InverterLUT Dict"=w310:T10)
        n131 = call <vilib>:"Easy Read XML File__JKI EasyXML.vi"("error in (no error)"=w302, "LabVIEW Data (Type)"=w297, "XML File Path"=w319) -> ("error out"=w307:errorcluster, "LabVIEW Data"=w308:variant)  [unwired: 6 in, 1 out]
        n132 = Variant To Data(error in=w307, type=w297, Variant=w308) -> (data=w309:T4, error out=w311:errorcluster)
        n133 = Unbundle(w309) -> ("Inverter Records"=w316:T5[])
        n134 = Array Size(array=w316) -> (size(s)=w317:i32)
        n135 = for {
          tunnel: w316 -> [w339] mode=indexing
          shift-right: [w340] -> w315
          shift-left: w311 -> [w341]
          shift-right: [w342] -> w314
          shift-left: w310 -> [w343]
          n136 = Unbundle By Name(w339) -> ("name"=w338:string)
          n137 = call <vilib>:"Set Dynamic CVT Data.vi"("error in (no error)"=w341, "value"=w339, "DataName"=w338, "dCVT DVR"=w343) -> ("error out"=w340:errorcluster, "dCVT DVR out"=w342:T10)  [unwired: 5 in, 1 out]
        }
        n138 = call <vilib>:"Get ALL Dynamic CVT Data.vi"("error in (no error)"=w315, "dCVT DVR"=w314) -> ("error out"=w304:errorcluster, "NameArray"=w303:string[], "ValueArray"=w305:variant[])  [unwired: 6 in, 1 out]
        n139 = for {
          tunnel: w305 -> [w328] mode=indexing
          tunnel: [w325] -> w296 mode=indexing
          shift-right: [w326] -> w301
          shift-left: w304 -> [w327]
          w324 = T5 {"name"="", "last updated"=timestamp(0 s since 1904-01-01), "type"="", "inverter Info"={"manufacturer"="", "model"="", "product"="", "serial"="", "power class"="", "year manf"=""}, "gain range"={"gain max"=0.0, "gain min"=0.0, "gain increment"=0.0}, "offset range"={"offset max"=0.0, "offset min"=0.0, "offset increment"=0.0}, "gain actual"=0.0, "offset actual"=0.0, "power level"=0.0, "minimum current"=0.0, "resistance single phase"=0.0, "resistance 3 phase"=0.0, "set flag"=0}  # CurrInverterRec
          n140 = Variant To Data(error in=w327, type=w324, Variant=w328) -> (data=w325:T5, error out=w326:errorcluster)
        }
        n141 = Array Size(array=w296) -> (size(s)=w322:i32)
        n142 = local write "Total"(w322) -> ()
        n143 = Not Equal?(x=w317, y=w322) -> (x != y?=w318:bool)
        n144 = Greater Than 0?(x=w322) -> (x > 0?=w312:bool)
        n145 = case shown="True" w312 {
          tunnel: ["" w335] -> w313
          tunnel: [0 ("CurrRec") 1 ("CurrRec")] -> w320
          tunnel: [-1 ("Inverter List") 0 ("Inverter List")] -> w321
          tunnel: w318 -> [_ w332]
          frame False {
          }
          frame True {
            n146 = case shown="True" w332 {
              tunnel: ["UI: Display Current Record" "UI: Warn Dup Records Eliminated"] -> w335
              frame False {
              }
              frame True {
              }
            }
          }
        }
        n147 = Index Array(array=w296) -> (element=w295:T5)  [unwired: 1 in]
        n148 = property on="Inverter List" class="LstBox (strict)"("Item Names"=w303) -> ()  [unwired: 2 in, 2 out]
        n149 = local write "CurrRec"(w320) -> ()
        n150 = local write "Inverter List"(w321) -> ()
        n151 = Bundle By Name(cluster=w306, "All Records"=w296, "CurrInverterRec"=w295) -> (w298:T11)
        n152 = call <vilib>:"Add State(s) to Queue__JKI_lib_State_Machine.vi"("State(s) in Front (\"\")"=w313, "State(s) in (\"\")"=w299) -> ("States Out"=w300:string)  [unwired: 13 in]
      }
      frame "Data: Initialize" {
        w346 = T5 {"name"="", "last updated"=timestamp(0 s since 1904-01-01), "type"="", "inverter Info"={"manufacturer"="", "model"="", "product"="", "serial"="", "power class"="", "year manf"=""}, "gain range"={"gain max"=0.0, "gain min"=0.0, "gain increment"=0.0}, "offset range"={"offset max"=0.0, "offset min"=0.0, "offset increment"=0.0}, "gain actual"=0.0, "offset actual"=0.0, "power level"=0.0, "minimum current"=0.0, "resistance single phase"=0.0, "resistance 3 phase"=0.0, "set flag"=0}  # CurrInverterRec
        (unwired) path ""  # Settings.Inverter Database File
        w352 = string[] []  # InverterNames[]
        w355 = T5[] []  # All Records
        w356 = T10 refnum  # InverterLUT Dict
        w359 = T12 {"Current VI Reference"=refnum, "Close Panel on Exit?"=FALSE}  # Core
        n153 = property class="Main.lvclass"(reference=w350) -> (reference out=w351:refnum<class "Main.lvclass">, "Accessors:InvLUTDict*"=w349:T10, "Accessors:ObjData*"=w348:T13)  [unwired: 1 in, 1 out]
        n154 = Unbundle By Name(w348) -> ("Settings.Inverter Database File"=w347:path)
        n155 = Get Date/Time In Seconds() -> (seconds since 1Jan1904=w344:timestamp)
        n156 = Bundle By Name(cluster=w346, "last updated"=w344) -> (w345:T5)
        n157 = local write "LUT File"(w347) -> ()
        n158 = Initialize Array(w345, 0 ("dimension size")) -> (w354:T5[])
        n159 = Variant To Data(type=w355, Variant=w354) -> (data=w358:T5[])  [unwired: 1 in, 1 out]
        n160 = property on="Inverter List" class="LstBox (strict)"("Item Names"=w352) -> ()  [unwired: 2 in, 2 out]
        n161 = Variant To Data(type=w356, Variant=w349) -> (data=w357:T10)  [unwired: 1 in, 1 out]
        n162 = Bundle("Core"=w359, "CurrInverterRec"=w345, "All Records"=w358, "Inverter Database File"=w347, "InverterLUT Dict"=w357) -> (w361:T11)  [unwired: 1 in]
        n163 = call <vilib>:"Add State(s) to Queue__JKI_lib_State_Machine.vi"("State(s) in (\"\")"=w363) -> ("States Out"=w362:string)  [unwired: 14 in]
      }
      frame "Data: Cleanup" {
        n164 = Unbundle By Name(w374) -> ("Inverter Database File"=w380:path, "InverterLUT Dict"=w381:T10, "Core.Current VI Reference"=w384:refnum<vi>)
        n165 = Unbundle By Name(w374) -> ("CurrInverterRec"=w373:T5)
        n166 = local read "LUT File"() -> (w377:path)
        n167 = Close Reference(reference=w384, error in (no error)=w383) -> (error out=w382:errorcluster)
        n168 = Not Equal?(x=w377, y=w380) -> (x != y?=w378:bool)
        n169 = Path To String(path=w377) -> (string=w375:string)
        n170 = property class="Main.lvclass"(reference=w379) -> (reference out=w370:refnum<class "Main.lvclass">, "Accessors:Settings*"=w372:T14)  [unwired: 1 in, 1 out]
        n171 = case shown="True" w378 {
          tunnel: w372 -> [w387 w390]
          tunnel: w377 -> [_ w389]
          tunnel: [w387 w388] -> w371
          frame False {
          }
          frame True {
            n172 = Bundle By Name(cluster=w390, "Inverter Database File"=w389) -> (w388:T14)
          }
        }
        n173 = Build Array(w373) -> (w364:T5[])
        n174 = property class="Main.lvclass"(reference=w370, "Accessors:Settings*"=w371, "Accessors:InvLUTDict*"=w381, "Accessors:CurrInverter*"=w364) -> (reference out=w366:refnum<class "Main.lvclass">, error out=w367:errorcluster)  [unwired: 1 in]
        n175 = call "Generate Async Cmd Event.vi"("error in (no error)"=w367, "AsyncCmd"=AsynCmd_Main--enum."Main.RefreshInverterList", "Main in"=w366) -> ("error out"=w368:errorcluster, "Main out"=w365:refnum<class "Main.lvclass">)  [unwired: 7 in]
        n176 = case shown="True" w378 {
          tunnel: "Notice: Inverter Database File has been changed in Main Settings memory, but\nthe configuration file has not been updated with the changed filename.\nIf you wish to make persistent the changed database filename,\nplease update the application's configuration file with desired Database Filename;\nnow using - \n[%s]" ("format string") -> [_ w392]
          tunnel: w375 -> [_ w391]
          tunnel: w368 -> [_ _]
          frame False {
          }
          frame True {
            w394 = ""
            n177 = Format Into String(format string=w392, w391) -> (resulting string=w395:string)  [unwired: 2 in, 1 out]
            n178 = call <vilib>:"Three Button Dialog.vi"("Window Title (\"\")"="**NOTICE **" ("Window Title (\"\")"), "Right Button Text (\"Cancel\")"=w394, "Center Button Text (\"No\")"="OK", "Left Button Text (\"Yes\")"=w394, "message"=w395) -> ()  [unwired: 6 in, 1 out]
          }
        }
        n179 = call <vilib>:"Add State(s) to Queue__JKI_lib_State_Machine.vi"("State(s) in (\"\")"=w386) -> ("States Out"=w385:string)  [unwired: 14 in]
      }
      frame "---------- UI ----------" {
        n180 = call <vilib>:"Add State(s) to Queue__JKI_lib_State_Machine.vi"("State(s) in (\"\")"=w401) -> ("States Out"=w400:string)  [unwired: 14 in]
      }
      frame "UI: Warn Dup Records Eliminated" {
        n181 = call <vilib>:"Three Button Dialog.vi"("Window Title (\"\")"="WARNING" ("Window Title (\"\")"), "Center Button Text (\"No\")"="", "message"="Warning: Some records had duplicate Inverter Names.\nInverter Names in the database must be unique.\n\nProceed to update database file with duplicate names removed?\n\nNote: \n<Cancel> terminates editor, and does not modify the database file.\n<Yes> Updates the database file with duplicate Inverter Name records eliminated.") -> ("Which Button?"=w403:T33)  [unwired: 8 in]
        n182 = case shown="\"Left Button\"" w403 {
          tunnel: ["Macro: Exit" "Data: Update Record\nUI: Display Current Record"] -> w402
          frame Default {
          }
          frame "Left Button" {
          }
        }
        n183 = call <vilib>:"Add State(s) to Queue__JKI_lib_State_Machine.vi"("State(s) in Front (\"\")"=w402, "State(s) in (\"\")"=w411) -> ("States Out"=w410:string)  [unwired: 13 in]
      }
      frame "UI: Display Current Record" {
        n184 = Unbundle By Name(w422) -> ("CurrInverterRec"=w421:T5)
        n185 = Unbundle By Name(w421) -> ("name"=w416:string, "last updated"=w415:timestamp, "type"=w433:string, "inverter Info"=w432:T3, "gain range"=w431:T2, "offset range"=w430:T1, "gain actual"=w429:dbl, "offset actual"=w428:dbl, "power level"=w426:dbl, "minimum current"=w427:dbl, "resistance single phase"=w425:dbl, "resistance 3 phase"=w424:dbl, "set flag"=w423:u16)
        n186 = property on="Inverter List" class="LstBox (strict)"() -> ("Item Names"=w420:string[])  [unwired: 2 in, 2 out]
        n187 = local write "inverter Info"(w432) -> ()
        n188 = local write "offset range"(w430) -> ()
        n189 = local write "offset actual"(w428) -> ()
        n190 = local write "minimum current"(w427) -> ()
        n191 = local write "resistance 3 phase"(w424) -> ()
        n192 = Search 1D Array(1D array=w420, element=w416) -> (index of element=w418:i32)  [unwired: 1 in]
        n193 = Format Date/Time String(seconds (now)=w415) -> (date/time string=w414:string)  [unwired: 2 in]
        n194 = local write "Inverter List"(w418) -> ()
        n195 = Increment(x=w418) -> (x+1=w419:i32)
        n196 = local write "name"(w416) -> ()
        n197 = local write "last updated"(w414) -> ()
        n198 = local write "type"(w433) -> ()
        n199 = local write "gain range"(w431) -> ()
        n200 = local write "gain actual"(w429) -> ()
        n201 = local write "power level"(w426) -> ()
        n202 = local write "resistance single phase"(w425) -> ()
        n203 = local write "set flag"(w423) -> ()
        n204 = local write "CurrRec"(w419) -> ()
        n205 = call <vilib>:"Add State(s) to Queue__JKI_lib_State_Machine.vi"("State(s) in (\"\")"=w436) -> ("States Out"=w435:string)  [unwired: 14 in]
      }
      frame "UI: Initialize" {
        n206 = Unbundle By Name(w444) -> ("CurrInverterRec"=w443:T5)
        n207 = Unbundle By Name(w443) -> ("name"=w456:string, "last updated"=w437:timestamp, "type"=w455:string, "inverter Info"=w454:T3, "gain range"=w453:T2, "offset range"=w452:T1, "gain actual"=w451:dbl, "offset actual"=w450:dbl, "power level"=w448:dbl, "minimum current"=w449:dbl, "resistance single phase"=w447:dbl, "resistance 3 phase"=w446:dbl, "set flag"=w445:u16)
        n208 = local write "Total"(0 ("Total")) -> ()
        n209 = local write "CurrRec"(0 ("CurrRec")) -> ()
        n210 = local write "name"(w456) -> ()
        n211 = local write "inverter Info"(w454) -> ()
        n212 = local write "offset range"(w452) -> ()
        n213 = local write "offset actual"(w450) -> ()
        n214 = local write "minimum current"(w449) -> ()
        n215 = local write "resistance 3 phase"(w446) -> ()
        n216 = local write "Inverter List"(-1 ("Inverter List")) -> ()
        n217 = Format Date/Time String(seconds (now)=w437) -> (date/time string=w438:string)  [unwired: 2 in]
        n218 = local write "last updated"(w438) -> ()
        n219 = local write "type"(w455) -> ()
        n220 = local write "gain range"(w453) -> ()
        n221 = local write "gain actual"(w451) -> ()
        n222 = local write "power level"(w448) -> ()
        n223 = local write "resistance single phase"(w447) -> ()
        n224 = local write "set flag"(w445) -> ()
        n225 = call <vilib>:"Add State(s) to Queue__JKI_lib_State_Machine.vi"("State(s) in (\"\")"=w459) -> ("States Out"=w458:string)  [unwired: 14 in]
      }
      frame "UI: OpenFrontPanel" {
        n226 = Unbundle By Name(w471) -> ("Core.Current VI Reference"=w470:refnum<vi>)
        n227 = invoke class="VI" method="FP.Open"(reference=w470, error in=w468, "Activate"=TRUE ("Activate?"), "State"=T9."Standard") -> (reference out=w469:refnum<vi>, error out=w477:errorcluster)  [unwired: 1 in, 3 out]
        n228 = call <userlib>:"MGI Get Executable Version.vi"() -> ("Version"=w464:string)  [unwired: 7 in]
        n229 = Format Into String(format string="Inverter LUT UI  [v%s]", w464) -> (resulting string=w463:string)  [unwired: 2 in, 1 out]
        n230 = property class="VI"(reference=w469, error in=w477, "FP.Behavior"=T7."Modal" ("Front Panel Window:Behavior")) -> (reference out=w466:refnum<vi>, error out=w476:errorcluster)
        n231 = property class="VI"(reference=w466, error in=w476, "Front Panel.Title"=w463) -> (error out=w467:errorcluster)  [unwired: 1 out]
        n232 = call <userlib>:"Fit VI window to Largest Dec__ogtk.vi"("error in (no error)"=w467, "border spacing (2 px)"=-2) -> ("error out"=w461:errorcluster)  [unwired: 4 in, 1 out]
        n233 = call <userlib>:"MGI Center Callee in Caller.vi"("Error In"=w461, "Caller VI Refnum (Callee's Caller)"="Caller VI Refnum (Callee's Caller)") -> ()  [unwired: 9 in, 1 out]
        n234 = call <vilib>:"Add State(s) to Queue__JKI_lib_State_Machine.vi"("State(s) in (\"\")"=w479) -> ("States Out"=w478:string)  [unwired: 14 in]
      }
      frame "UI: Cursor Set" {
        # "Argument"
        n235 = case shown="\"Idle\", Default" w481 {
          tunnel: w483 -> [w488 w490]
          tunnel: [w487 w489] -> w482
          frame "Idle", Default {
            n236 = call <vilib>:"Unset Busy.vi"("error in (no error)"=w488) -> ("error out"=w487:errorcluster)  [unwired: 10 in]
          }
          frame "Busy" {
            n237 = call <vilib>:"Set Busy.vi"("error in (no error)"=w490) -> ("error out"=w489:errorcluster)  [unwired: 9 in, 1 out]
          }
        }
        n238 = call <vilib>:"Add State(s) to Queue__JKI_lib_State_Machine.vi"("State(s) in (\"\")"=w486) -> ("States Out"=w485:string)  [unwired: 14 in]
      }
      frame "UI: Front Panel State" {
        # "Use other cases for open/close front panel"
        # "Argument"
        n239 = Unbundle By Name(w494) -> ("Core.Current VI Reference"=w493:refnum<vi>)
        n240 = case shown="\"Open\", Default" w492 {
          tunnel: w496 -> [w502 w515]
          tunnel: [w504 w516] -> w495
          tunnel: w493 -> [w503 w513]
          frame "Open", Default {
            n241 = property class="VI"(reference=w503, error in=w502) -> (reference out=w500:refnum<vi>, error out=w501:errorcluster, "Front Panel.Open"=w499:bool)
            n242 = case shown="False" w499 {
              tunnel: [w507 w510] -> w504
              tunnel: w501 -> [w506 w510]
              tunnel: w500 -> [w505 _]
              frame False {
                n243 = invoke class="VI" method="FP.Open"(reference=w505, error in=w506, "Activate"=TRUE, "State"=T9."Standard") -> (error out=w507:errorcluster)  [unwired: 1 in, 4 out]
              }
              frame True {
              }
            }
          }
          frame "Close" {
            n244 = property class="VI"(reference=w513, error in=w515) -> (reference out=w512:refnum<vi>, error out=w514:errorcluster, "Front Panel.Open"=w511:bool)
            n245 = case shown="True" w511 {
              tunnel: [w517 w520] -> w516
              tunnel: w514 -> [w517 w519]
              tunnel: w512 -> [_ w518]
              frame False {
              }
              frame True {
                n246 = invoke class="VI" method="FP.Close"(reference=w518, error in=w519) -> (error out=w520:errorcluster)  [unwired: 1 in, 2 out]
              }
            }
          }
        }
        n247 = call <vilib>:"Add State(s) to Queue__JKI_lib_State_Machine.vi"("State(s) in (\"\")"=w498) -> ("States Out"=w497:string)  [unwired: 14 in]
      }
      frame "---------- Macro ----------" {
        n248 = call <vilib>:"Add State(s) to Queue__JKI_lib_State_Machine.vi"("State(s) in (\"\")"=w525) -> ("States Out"=w524:string)  [unwired: 14 in]
      }
      frame "Macro: Initialize" {
        n249 = call <vilib>:"Add State(s) to Queue__JKI_lib_State_Machine.vi"("State(s) in Front (\"\")"=w527, "State(s) in (\"\")"=w531) -> ("States Out"=w530:string)  [unwired: 13 in]
      }
      frame "Macro: Exit" {
        n250 = Unbundle By Name(w539) -> ("Core.Close Panel on Exit?"=w538:bool)
        n251 = Select(t="// UI: Front Panel State >> Close", s=w538, f="") -> (s? t:f=w535:string)
        n252 = call <vilib>:"Add State(s) to Queue__JKI_lib_State_Machine.vi"("State(s) in (\"\")"=w535, "State(s) at Back (\"\")"=w533) -> ("States Out"=w534:string)  [unwired: 13 in]
        n253 = call <vilib>:"Add State(s) to Queue__JKI_lib_State_Machine.vi"("State(s) in Front (\"\")"=w534, "State(s) in (\"\")"=w542) -> ("States Out"=w541:string)  [unwired: 13 in]
      }
      frame "---------- Action ----------" {
        n254 = call <vilib>:"Add State(s) to Queue__JKI_lib_State_Machine.vi"("State(s) in (\"\")"=w547) -> ("States Out"=w546:string)  [unwired: 14 in]
      }
    }
  }
  "Main out" <- w1
